vi "Differential_delay_line_configuration_Mezzaninev56_initialize.vi"(0 "error in (no error)":errorcluster) -> (2 "error out 2":errorcluster)   [LabVIEW 2012]
panel:
  out "data out serial":string
  out "hex integer string":string
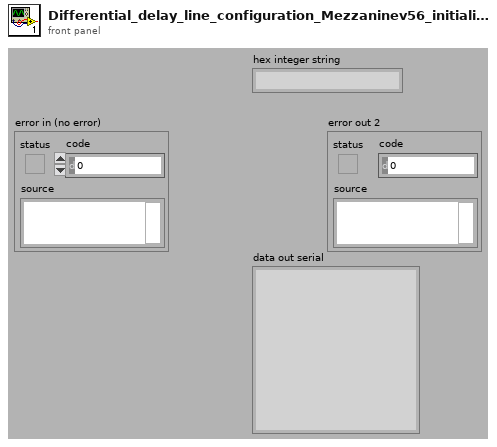
[diagram p1: front panel]
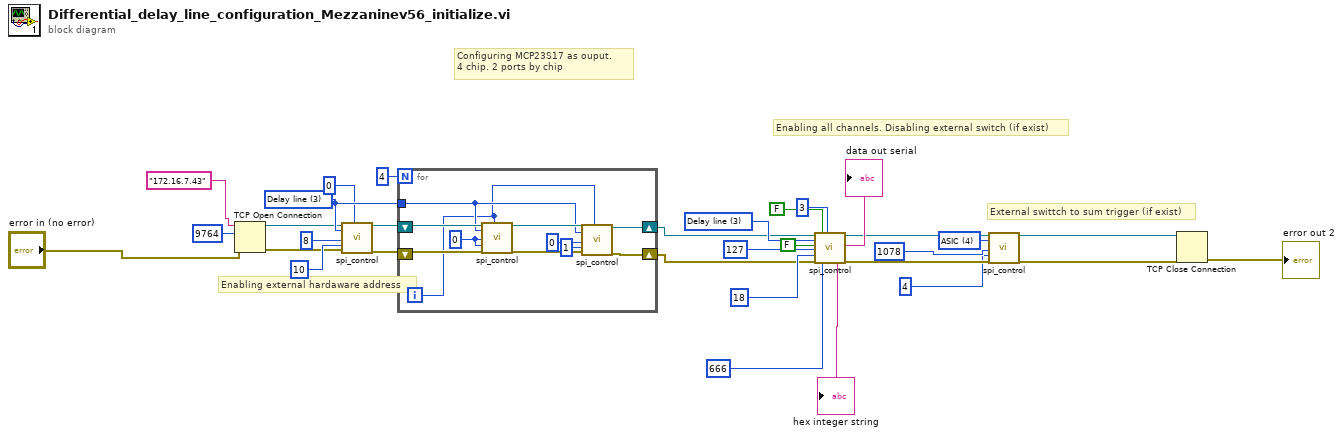
[diagram p0: block diagram]
diagram:
  w3 = u16 4 items=["Attenuation", "Clipping", "Enable channel", "Delay line", "ASIC"] ("Device")
  w28 = u16 3 items=["Attenuation", "Clipping", "Enable channel", "Delay line", "ASIC"] ("Device")
  w20 = u16 3 items=["Attenuation", "Clipping", "Enable channel", "Delay line", "ASIC"] ("Device")
  # "External swittch to sum trigger (if exist)"
  # "Enabling external hardaware address"
  # "Configuring MCP23S17 as ouput.\n4 chip. 2 ports by chip"
  # "Enabling all channels. Disabling external switch (if exist)"
  n1 = TCP Open Connection(address="172.16.7.43", remote port or service name=u16 9764, error in (no error)="error in (no error)") -> (connection ID=w19:refnum<k5>, error out=w16:errorcluster)  [unwired: 2 in]
  n2 = call "spi_control.vi"("connection ID"=w19, "Device"=w20, "Data"=8, "Register or channel"=10, "error out 3"=w16, "chip delay"=0) -> ("connection ID out"=w18:refnum<k5>, "error out 2"=w17:errorcluster)  [unwired: 6 in, 6 out]
  n3 = for {
    N: 4 -> [_]
    tunnel: w20 -> [w36]
    shift-right: [w42] -> w25
    shift-left: w17 -> [w40]
    shift-right: [w37] -> w24
    shift-left: w18 -> [w39]
    i -> [w32]
    w34 = 0 ("Data")
    n4 = call "spi_control.vi"("connection ID"=w39, "Device"=w36, "Data"=w34, "Register or channel"=w34, "error out 3"=w40, "chip delay"=w32) -> ("connection ID out"=w38:refnum<k5>, "error out 2"=w41:errorcluster)  [unwired: 6 in, 6 out]
    n5 = call "spi_control.vi"("connection ID"=w38, "Device"=w36, "Data"=0, "Register or channel"=1, "error out 3"=w41, "chip delay"=w32) -> ("connection ID out"=w37:refnum<k5>, "error out 2"=w42:errorcluster)  [unwired: 6 in, 6 out]
  }
  n6 = call "spi_control.vi"("connection ID"=w24, "Device"=w28, "Read/#write"=FALSE, "Data"=127, "Register or channel"=18, "error out 3"=w25, "Read physical"=FALSE, "Id in"=666, "chip delay"=3 ("Channel delay")) -> ("hex integer string"=→"hex integer string":string, "connection ID out"=w4:refnum<k5>, "data out serial"=→"data out serial":string, "error out 2"=w5:errorcluster)  [unwired: 3 in, 4 out]
  n7 = call "spi_control.vi"("connection ID"=w4, "Device"=w3, "Data"=1078, "Register or channel"=4, "error out 3"=w5) -> ("connection ID out"=w7:refnum<k5>, "error out 2"=w6:errorcluster)  [unwired: 7 in, 6 out]
  n8 = TCP Close Connection(connection ID=w7, error in (no error)=w6) -> (error out=→"error out 2":errorcluster)  [unwired: 1 in, 1 out]
